vi "Find bad code.vi"() -> ()   [LabVIEW 2024]
panel:
  in  "Continue":bool
  in  "Open bad":bool=TRUE
  in  "Stop on bad":bool=TRUE
  out "Execution:State":T1(ring)
  out "Bad files":path[](array[path])
  in  "Stop Button":bool
  out "File Path":path
  out "Progress":string
  in  "Folder Path":path
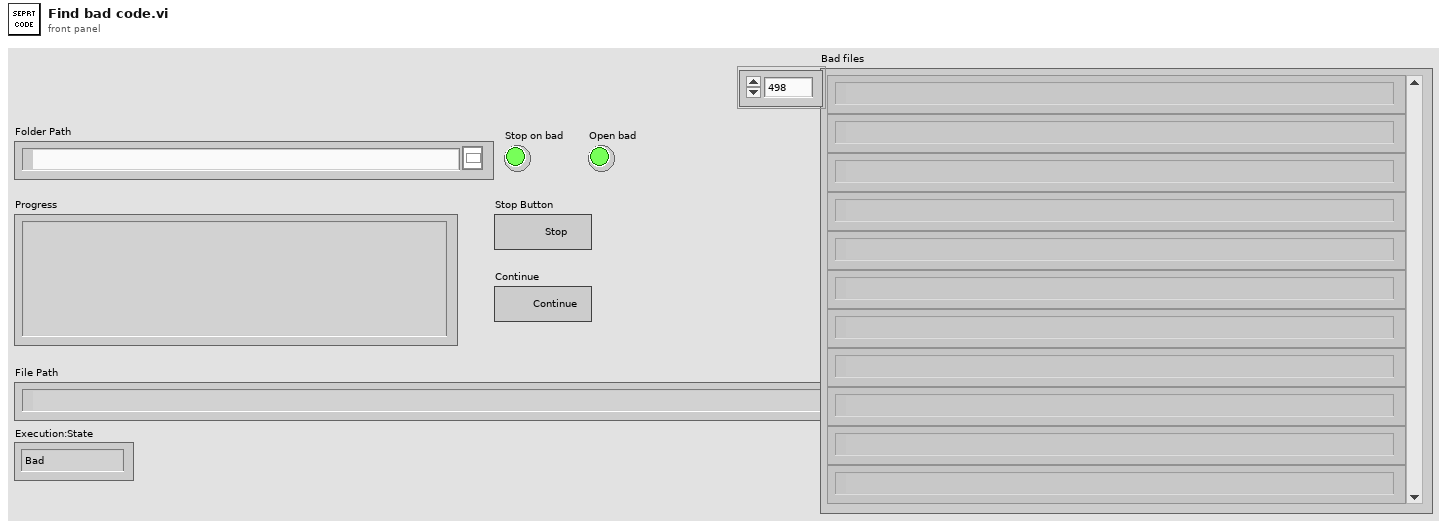
[diagram p1: front panel]
types:
  T1 = enum32{"Bad", "Idle", "Run top level", "Running"}
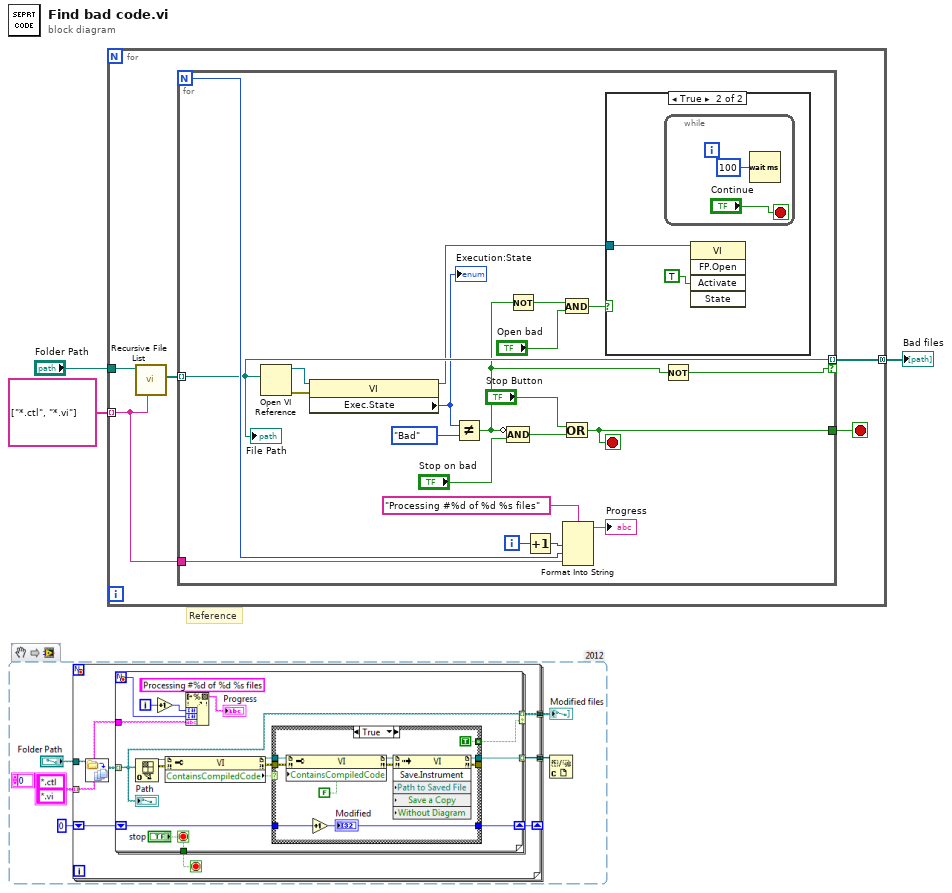
[diagram p0: block diagram]
diagram:
  # "Reference"
  n1 = for {
    tunnel: string[] ["*.ctl", "*.vi"] -> [w6] mode=indexing
    tunnel: "Folder Path" -> [w8]
    tunnel: [w4] -> w1 mode=concatenating
    stop <- w5 stop-if-true
    n2 = call <vilib>:"Recursive File List.vi"("pattern"=w6, "Folder Path"=w8) -> ("All Files in Dir"=w7:path[])  [unwired: 5 in, 4 out]
    n3 = for {
      N -> [w26]
      tunnel: w7 -> [w20] mode=indexing
      tunnel: w6 -> [w25]
      tunnel: [w16] -> w5
      tunnel: [w20] -> w4 mode=indexing if=w14
      i -> [w28]
      stop <- w16 stop-if-true
      n4 = Open VI Reference(vi path=w20) -> (vi reference=w23:refnum<vi>, error out=w22:errorcluster)  [unwired: 5 in]
      n5 = property class="VI"(reference=w23, error in=w22) -> (reference out=w9:refnum<vi>, "Exec.State"=w19:T1)  [unwired: 1 out]
      "Execution:State" <- w19
      n6 = Not Equal?(x=w19, y=T1."Bad" ("Execution:State")) -> (x != y?=w10:bool)
      n7 = Compound Arithmetic op=AND(invert w10, "Stop on bad") -> (w15:bool)
      n8 = Not(x=w10) -> (.not. x?=w13:bool)
      n9 = Increment(x=w28) -> (x+1=w27:i32)
      n10 = And(x=w13, y="Open bad") -> (x .and. y?=w11:bool)
      n11 = Or(x="Stop Button", y=w15) -> (x .or. y?=w16:bool)
      n12 = Format Into String(format string="Processing #%d of %d %s files", w27, w26, w25) -> (resulting string=→"Progress":string)  [unwired: 2 in, 1 out]
      n13 = case shown="True" w11 {
        tunnel: w9 -> [_ w31]
        frame False {
        }
        frame True {
          n14 = while {
            stop <- "Continue" stop-if-true
            n15 = Wait (ms)(milliseconds to wait=u32 100) -> ()  [unwired: 1 out]
          }
          n16 = invoke class="VI" method="FP.Open"(reference=w31, "Activate"=TRUE ("Activate?")) -> ()  [unwired: 3 in, 5 out]
        }
      }
      n17 = Not(x=w10) -> (.not. x?=w14:bool)
      "File Path" <- w20
    }
  }
  "Bad files" <- w1
